vi "Pulse Slow-Fast (Set).vi"(6 "ISOBUS address":T3=-1 caption="ISOBUS address (-1)", 8 "error in":errorcluster, 10 "Delay":string caption="SLOW_ON/OFF", 11 "Mercury Reference In":T4) -> (0 "error out":errorcluster, 2 "Response":T1, 3 "Mercury Reference Out":T4, 4 "Valid?":T2)   [LabVIEW 2013, in "Mercury iXX.lvlib" / "Level Meter.lvlib"]
doc: "Set the current delay of the helium pulse."
uses:
  <instrlib>/Mercury iXX/Public/Libraries/Level Meter.lvlib
  <instrlib>/Mercury iXX/Public/Controls/Mercury Reference.ctl
  <instrlib>/Mercury iXX/Public/Controls/Comms Transport Layer.ctl
  <instrlib>/Mercury iXX/Private/Controls/Query Dynamic Reference.ctl
  <instrlib>/Mercury iXX/Public/Controls/ISOBus Address.ctl
  <instrlib>/Mercury iXX/Public/Controls/Is Valid LED.ctl
  <instrlib>/Mercury iXX/Public/Controls/Response String.ctl
  <instrlib>/Mercury iXX/Private/Controls/Command Verbs.ctl
  <instrlib>/Mercury iXX/Mercury iXX.lvlib
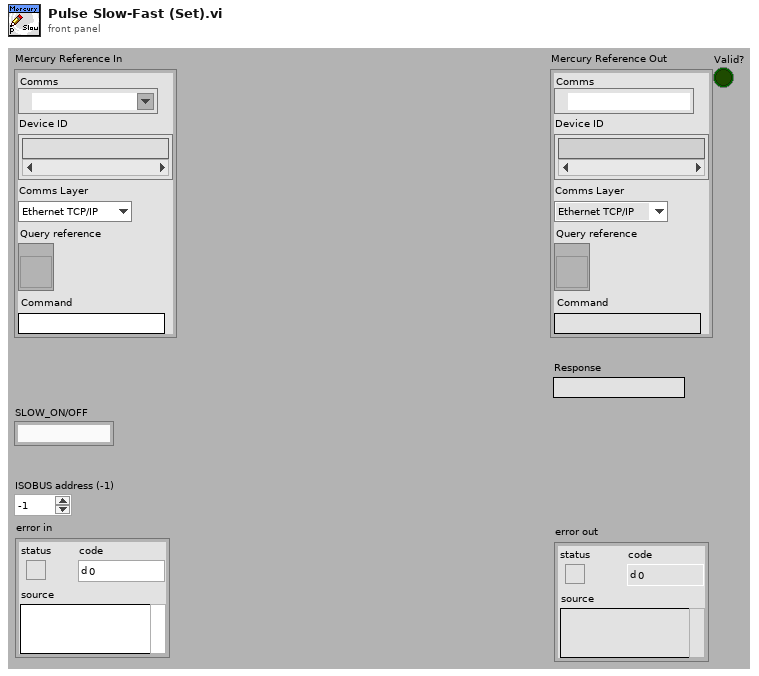
[diagram p1: front panel]
types:
  T1 = typedef "Mercury iXX.lvlib/Response String.ctl" = string
  T2 = typedef "Mercury iXX.lvlib/Is Valid LED.ctl" = bool
  T3 = typedef "Mercury iXX.lvlib/ISOBus Address.ctl" = i32
  T4 = typedef "Mercury iXX.lvlib/Mercury Reference.ctl" = cluster{"Comms":refnum<visa-resource-name>, "Device ID":string[], "Comms Layer":T5, "Command":string, "Query reference":T6}
  T5 = typedef "Mercury iXX.lvlib/Comms Transport Layer.ctl" = enum16{"Ethernet TCP/IP", "USB", "ISOBus - RS-232", "GPIB"}
  T6 = typedef "Mercury iXX.lvlib/Query Dynamic Reference.ctl" = refnum<vi>
  T7 = typedef "Mercury iXX.lvlib/Command Verbs.ctl" = string
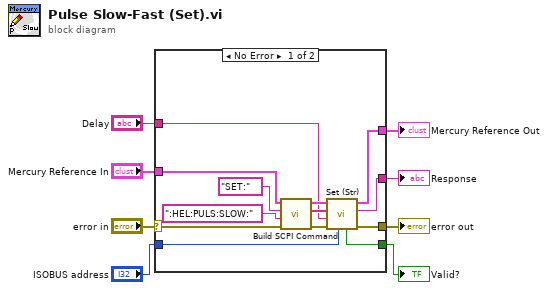
[diagram p0: block diagram]
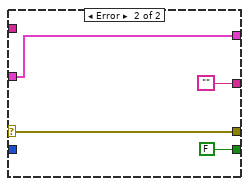
[diagram p2: hidden frame]
diagram:
  n1 = case shown="No Error" "error in" {
    selector: "error in" -> [w20 w24]
    tunnel: "Mercury Reference In" -> [w21 w25]
    tunnel: "ISOBUS address" -> [w13 _]
    tunnel: [w12 T2 FALSE ("Valid?")] -> w2
    tunnel: [w10 ""] -> w3
    tunnel: [w9 w25] -> w4
    tunnel: "Delay" -> [w15 _]
    tunnel: [w11 w24] -> w1
    frame No Error {
      n2 = call <instrlib>:"Build SCPI Command.vi"("error in"=w20, "Noun(s)"=":HEL:PULS:SLOW:" ("Command"), "Verb"=T7 "SET:", "Mercury Reference In"=w21) -> ("error out"=w14:errorcluster, "SCPI Message(s)"=w16:string[], "Mercury Reference Out"=w17:T4)  [unwired: 5 out]
      n3 = call <instrlib>:"Set (Str).vi"("ISOBUS address"=w13, "error in"=w14, "Command Value (Str)"=w15, "SCPI Message(s)"=w16, "Mercury Reference In"=w17) -> ("error out"=w11:errorcluster, "Response"=w10:T1, "Mercury Reference Out"=w9:T4, "Valid?"=w12:T2)  [unwired: 3 out]
    }
    frame Error {
    }
  }
  "Mercury Reference Out" <- w4
  "Valid?" <- w2
  "error out" <- w1
  "Response" <- w3
